vi "Zero Measured Flow Rate.vi"(8 "error in (no error)":errorcluster, 11 "RRG in":refnum<class "PL Eltochpribor RRG.lvclass">) -> (0 "error out":errorcluster, 3 "RRG out":refnum<class "PL Eltochpribor RRG.lvclass">)   [LabVIEW 2015, in "PL Eltochpribor RRG.lvclass"]
doc: "Sets current measured flow rate as zero."
uses:
  PL Eltochpribor RRG.lvclass
  <vilib>/plasmapper/PL Modbus Client/PL Modbus Client.lvclass
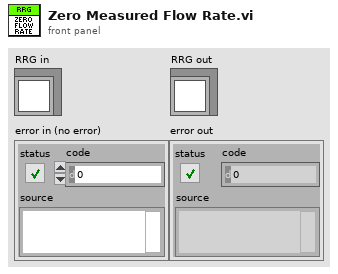
[diagram p1: front panel]
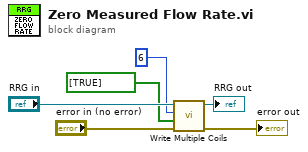
[diagram p0: block diagram]
diagram:
  n1 = call <vilib>:"Write Multiple Coils.vi"("error in (no error)"="error in (no error)", "values"=bool[] [TRUE] ("value"), "address"=u16 6, "MODBUS in"="RRG in") -> ("error out"=→"error out":errorcluster, "MODBUS out"=→"RRG out":refnum<class "PL Eltochpribor RRG.lvclass">)  [unwired: 6 in]
